vi "PASCO_PID.vi"(0 "Delta":dbl(slide) scale=0.0..1.0, 9 "Integral Reset":bool, 11 "Deadband":dbl=0.001, 12 "P Gain":dbl=1.0, 13 "I Gain":dbl, 14 "D Gain":dbl) -> (4 "Output":dbl, 10 "IsThere":bool)   [LabVIEW 2013]
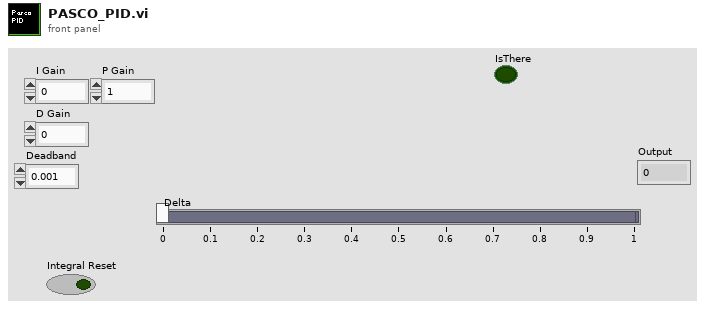
[diagram p1: front panel]
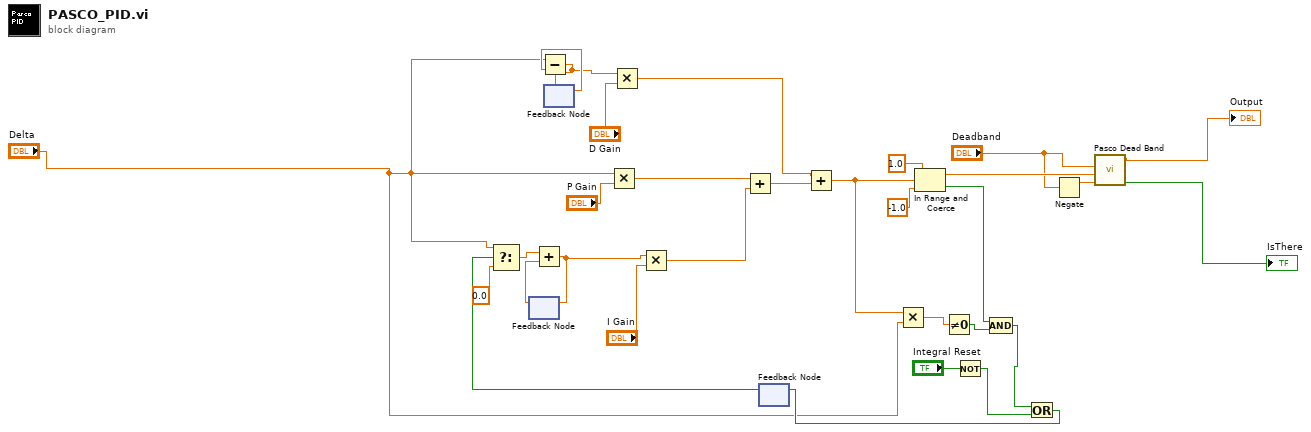
[diagram p0: block diagram]
diagram:
  n1 = feedback #1() -> (w27:dbl)  [unwired: 1 in]
  n2 = feedback #2() -> (w26:dbl)  [unwired: 1 in]
  n3 = Subtract(x="Delta", y=w26) -> (x-y=w25:dbl)
  n4 = feedback-in #2(w25) -> ()
  n5 = Multiply(x="Delta", y="P Gain") -> (x*y=w9:dbl)
  n6 = Multiply(x=w25, y="D Gain") -> (x*y=w18:dbl)
  n7 = feedback #3() -> (w12:bool)  [unwired: 1 in]
  n8 = Select(t="Delta", s=w12, f=0.0) -> (s? t:f=w19:dbl)
  n9 = Add(x=w19, y=w27) -> (x+y=w10:dbl)
  n10 = feedback-in #1(w10) -> ()
  n11 = Multiply(x=w10, y="I Gain") -> (x*y=w8:dbl)
  n12 = Add(x=w9, y=w8) -> (x+y=w17:dbl)
  n13 = Add(x=w18, y=w17) -> (x+y=w16:dbl)
  n14 = Multiply(x=w16, y="Delta") -> (x*y=w23:dbl)
  n15 = In Range and Coerce(upper limit=1.0, x=w16, lower limit=-1.0) -> (coerced(x)=w15:dbl, In Range?=w21:bool)
  n16 = Not Equal To 0?(x=w23) -> (x != 0?=w22:bool)
  n17 = Not(x="Integral Reset") -> (.not. x?=w5:bool)
  n18 = Compound Arithmetic op=AND(w21, w22) -> (w6:bool)
  n19 = Or(x=w6, y=w5) -> (x .or. y?=w4:bool)
  n20 = feedback-in #3(w4) -> ()
  n21 = Negate(x="Deadband") -> (-x=w14:dbl)
  n22 = call "Pasco Dead Band.vi"("lower limit"=w14, "PWM Power"=w15, "upper limit"="Deadband") -> ("Integral Reset"=→"IsThere":bool, "PWM Power"=→"Output":dbl)  [unwired: 7 in]
